vi "pwrite flush serial.vi"(11 "resourceId":i32) -> (3 "resourceId out":i32)   [LabVIEW 2010, in "libcommon_serial.lvlib"]
doc: "clean the outcoming write buffer\n\nvoid pwrite_flush_serial(pserial_handle_t h);"
uses:
  <userlib>/libcommon_serial/libcommon_serial.lvlib
  <userlib>/libcommon_serial/libcommon_serial.so
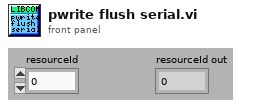
[diagram p1: front panel]
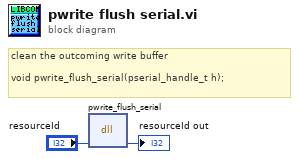
[diagram p0: block diagram]
diagram:
  # "clean the outcoming write buffer\n\nvoid pwrite_flush_serial(pserial_handle_t h);"
  n1 = dll-call lib="usr/local/natinst/LabVIEW-2010/user.lib/libcommon_serial/libcommon_serial.*" fn="pwrite_flush_serial"("resourceId"="resourceId") -> ("resourceId"=→"resourceId out":i32)  [unwired: 4 in, 2 out]
